vi "Sim Read DI DAQ Data.vi"(0 "DaqDevice dCVT":T1, 1 "DI TaskName":string, 5 "DaqData dCVT":T1, 7 "DI IONames":string[](array[string]), 11 "error in":errorcluster) -> (4 "DaqDevice dCVT out":T1, 6 "DaqData dCVT out":T1, 15 "error out":errorcluster)   [LabVIEW 2017, in "DAQ.lvclass"]
doc: "Developed by Kevin Thompson\nkevin@thompsonengineering.net\n\nCopyright 2018-2020\nThompson Engineering, LLC"
uses:
  DAQ.lvclass
  <vilib>/TELLC/Dynamic CVT API/TD Dynamic CVT DVR--ref.ctl
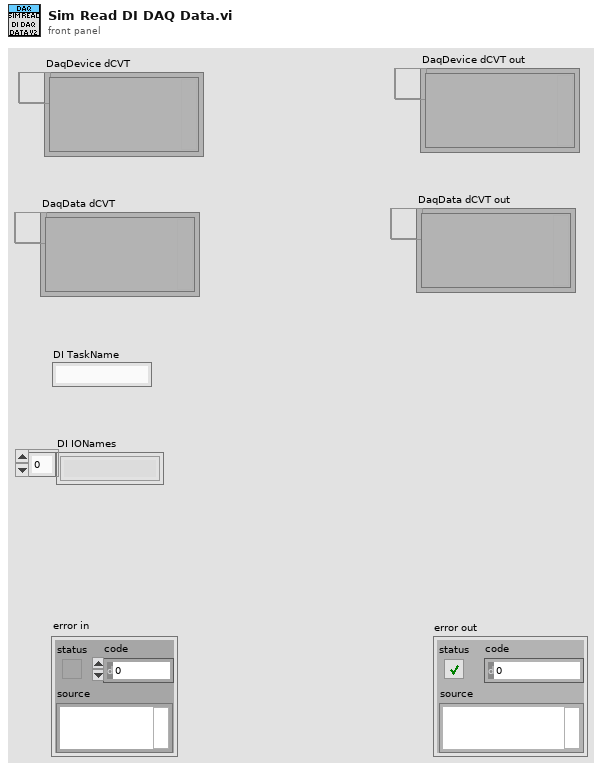
[diagram p1: front panel]
types:
  T1 = typedef "TD Dynamic CVT DVR--ref.ctl" = refnum<data-value>
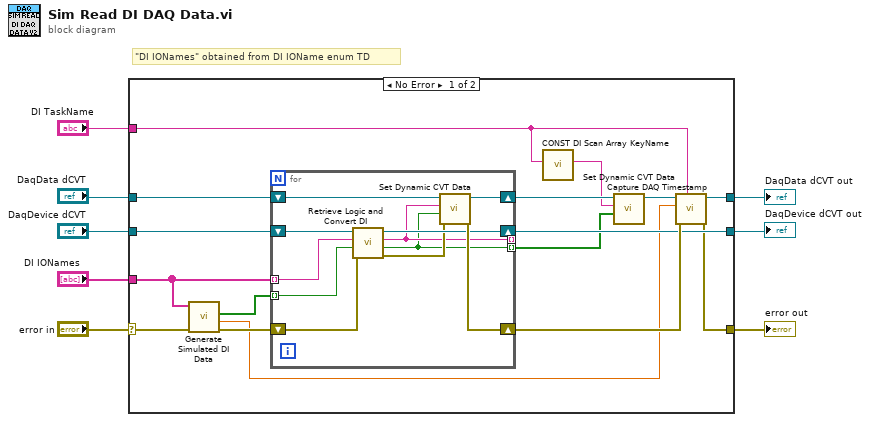
[diagram p0: block diagram]
diagram:
  # "\"DI IONames\" obtained from DI IOName enum TD"
  n1 = case shown="No Error" "error in" {
    selector: "error in" -> [w19 w37]
    tunnel: "DI TaskName" -> [w10 _]
    tunnel: "DI IONames" -> [w15 _]
    tunnel: "DaqData dCVT" -> [w24 w38]
    tunnel: [w23 w38] -> w2
    tunnel: [w11 w37] -> w3
    tunnel: "DaqDevice dCVT" -> [w21 w36]
    tunnel: [w20 w36] -> w1
    frame No Error {
      n2 = call "Generate Simulated DI Data.vi"("error in"=w19, "IONames[]"=w15) -> ("error out"=w17:errorcluster, "timestamp"=w16:dbl, "data"=w18:bool[])  [unwired: 7 in]
      n3 = for {
        tunnel: w18 -> [w28] mode=indexing
        tunnel: w15 -> [w27] mode=indexing
        shift-right: [w34] -> w14
        shift-left: w24 -> [w35]
        shift-right: [w33] -> w22
        shift-left: w17 -> [w30]
        shift-right: [w31] -> w20
        shift-left: w21 -> [w32]
        tunnel: [w26] -> _ mode=indexing
        tunnel: [w25] -> w12 mode=indexing
        n4 = call "Retrieve Logic and Convert DI.vi"("error in (no error)"=w30, "RawValue in"=w28, "IOName"=w27, "DAQ Node Dict DVR"=w32) -> ("error out"=w29:errorcluster, "ConvertedValue Out"=w25:bool, "IOName out"=w26:string, "DAQ Node Dict DVR out"=w31:T1)  [unwired: 4 in]
        n5 = call <vilib>:"Set Dynamic CVT Data.vi"("error in (no error)"=w29, "value"=w25, "DataName"=w26, "dCVT DVR"=w35) -> ("error out"=w33:errorcluster, "dCVT DVR out"=w34:T1)  [unwired: 5 in, 1 out]
      }
      n6 = call "CONST DI Scan Array KeyName.vi"("DI TaskName"=w10) -> ("DI ScanArray (KeyName)"=w9:string)  [unwired: 10 in]
      n7 = call <vilib>:"Set Dynamic CVT Data.vi"("value"=w12, "DataName"=w9, "dCVT DVR"=w14) -> ("dCVT DVR out"=w13:T1)  [unwired: 6 in, 2 out]
      n8 = call "Capture DAQ Timestamp.vi"("DaqData dCVT"=w13, "timestamp in"=w16, "error in (no error)"=w22, "AI TaskName"=w10) -> ("DaqData dCVT out"=w23:T1, "error out"=w11:errorcluster)  [unwired: 4 in, 1 out]
    }
    frame Error {
    }
  }
  "DaqData dCVT out" <- w2
  "error out" <- w3
  "DaqDevice dCVT out" <- w1
